vi "Write Error Action.vi"(8 "error in (no error)":errorcluster, 10 "Error Action":T1=enum."Ignore Error and Close Sink", 11 "Log Sink in":refnum<class "Log Sink.lvclass">) -> (0 "error out":errorcluster, 3 "Log Sink out":refnum<class "Log Sink.lvclass">)   [LabVIEW 2020, in "MVA Framework.lvlib" / "Composed Log.lvlib" / "Log Sink.lvclass"]
uses:
  Log Sink.lvclass
  Sink Error Actions ENUM.ctl
  Log Sink.lvclass/Log Sink.ctl
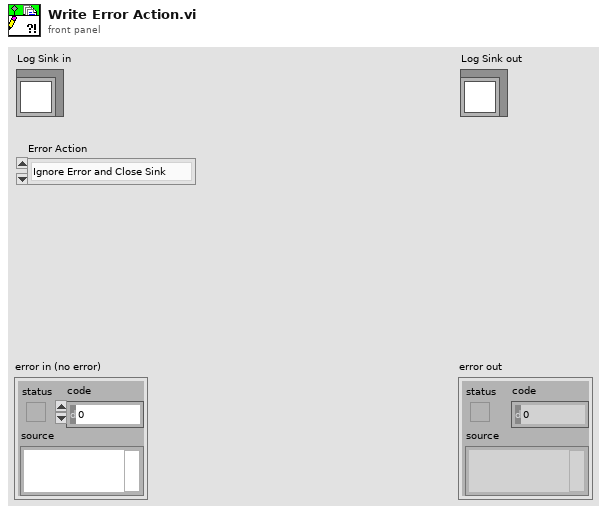
[diagram p1: front panel]
types:
  T1 = typedef "MVA Framework.lvlib/Composed Log.lvlib/Log Sink.lvclass/Sink Error Actions ENUM.ctl" = enum16{"Ignore Error and Continue", "Ignore Error and Close Sink", "Report Error and Close Sink"}
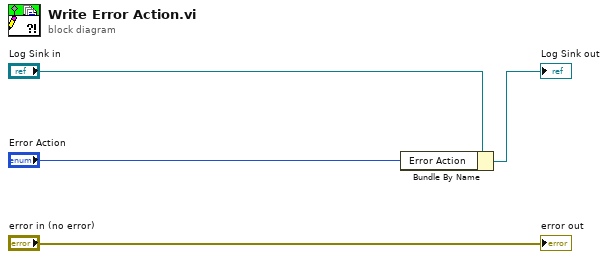
[diagram p0: block diagram]
diagram:
  n1 = Bundle By Name(cluster="Log Sink in", "Error Action"="Error Action") -> (→"Log Sink out":refnum<class "Log Sink.lvclass">)
  "error out" <- "error in (no error)"
